vi "pushButton.vi"(8 "error in (no error)":errorcluster, 10 "Button":T1, 11 "Inst.FP":refnum<class "Inst.FP.lvclass">) -> (0 "error out":errorcluster, 3 "Inst.FP out":refnum<class "Inst.FP.lvclass">)   [LabVIEW 2019, in "Inst.FP.lvclass"]
doc: "Programmatically pushes buttons on the Leiden GHS. The following buttons are supported: Start, 3He, 4He, Normal, Recovery, Auto, LED Test, and Reset.\n\n<b>Note</b>: some buttons do nothing by themselves but instead require a sequence of buttons to change modes. The API \"Set Mode\" takes care of this sequencing for you."
uses:
  Inst.FP.lvclass
  C:/Program Files (x86)/National Instruments/LabVIEW 2019/user.lib/LevyLab/Instrument Framework/Instrument/Instrument.lvclass
  Typedefs/Inst.FP.Buttons--Enum.ctl
  Typedefs/Inst.FP.Commands--Enum.ctl
  Typedefs/Inst.FP.pushButton--Cluster.ctl
  <userlib>/LevyLab/Instrument Framework/Instrument/Instrument.lvclass
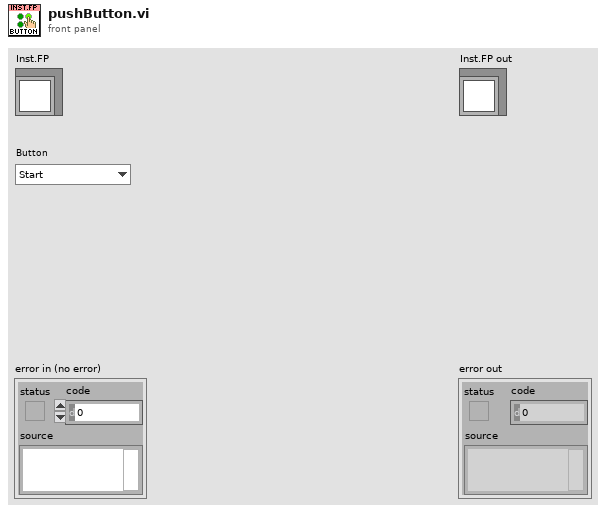
[diagram p1: front panel]
types:
  T1 = typedef "Inst.FP.lvclass/Inst.FP.Buttons--Enum.ctl" = enum16{"Start", "3He", "4He", "Normal", "Recovery", "Auto", "LED Test", "Reset"}
  T2 = typedef "Inst.FP.lvclass/Inst.FP.pushButton--Cluster.ctl" = cluster{"Button":T1}
  T3 = typedef "Inst.FP.lvclass/Inst.FP.Commands--Enum.ctl" = enum16{"getMode", "setMode", "pushButton"}
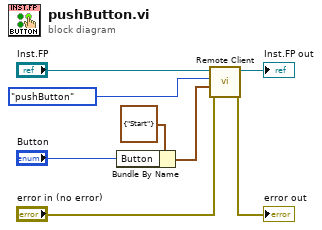
[diagram p0: block diagram]
diagram:
  n1 = Bundle By Name(cluster=T2 {"Button"=enum."Start"} ("Push Button"), "Button"="Button") -> (w3:T2)
  n2 = call <userlib>:"Remote Client.vi"("error in (no error)"="error in (no error)", "Data in"=w3, "Command in"=Inst.FP.Commands--Enum."pushButton" ("Commands"), "Instrument in"="Inst.FP") -> ("error out"=→"error out":errorcluster, "Instrument out"=→"Inst.FP out":refnum<class "Inst.FP.lvclass">)  [unwired: 4 in, 2 out]
